vi "Wait for Acquisition Complete.vi"(8 "error in (no error)":errorcluster, 10 "Maximum Time (10000 ms)":i32=10000, 11 "VISA resource name":refnum<visa-resource-name>) -> (0 "error out":errorcluster, 3 "VISA resource name out":refnum<visa-resource-name>)   [LabVIEW 2018, in "Agilent U2000 Series.lvlib"]
doc: "Waits for the current acquisition to finish. This VI should be called after Initiate VI and before Fetch VI.\n\nNote:\nUse this VI only with other low-level VIs. The high-level VIs automatically incorporate this functionality. This VI does not check the instrument status."
uses:
  Agilent U2000 Series.lvlib
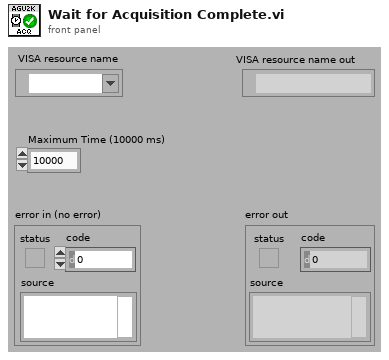
[diagram p1: front panel]
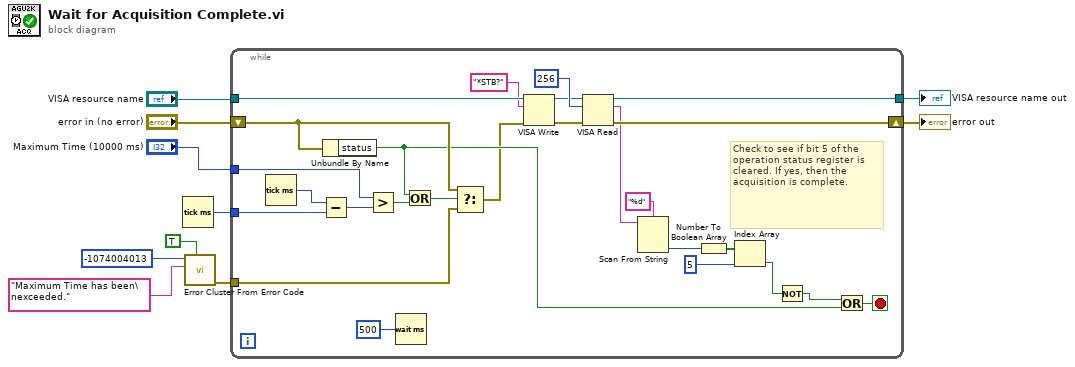
[diagram p0: block diagram]
diagram:
  n1 = Tick Count (ms)() -> (millisecond timer value=w4:u32)
  n2 = call <vilib>:"Error Cluster From Error Code.vi"("show call chain? (False)"=TRUE, "error message (\"\")"="Maximum Time has been\nexceeded." ("error message (\"\")"), "error code (0)"=-1074004013) -> ("error out"=w3:errorcluster)  [unwired: 1 in, 5 out]
  n3 = while {
    tunnel: [w35] -> w1
    tunnel: "VISA resource name" -> [w19]
    tunnel: "Maximum Time (10000 ms)" -> [w31]
    tunnel: w4 -> [w32]
    tunnel: w3 -> [w27]
    shift-right: [w36] -> w2
    shift-left: "error in (no error)" -> [w28]
    stop <- w26 stop-if-true
    # "Check to see if bit 5 of the operation status register is cleared. If yes, then the acquisition is complete."
    n4 = Tick Count (ms)() -> (millisecond timer value=w34:u32)
    n5 = Subtract(x=w34, y=w32) -> (x-y=w33:u32)
    n6 = Unbundle By Name(w28) -> ("status"=w25:bool)
    n7 = Greater?(x=w31, y=w33) -> (0:w30:bool)
    n8 = Wait (ms)(milliseconds to wait=u32 500) -> ()  [unwired: 1 out]
    n9 = Or(x=w25, y=w30) -> (x .or. y?=w29:bool)
    n10 = Select(t=w28, s=w29, f=w27) -> (s? t:f=w20:errorcluster)
    n11 = VISA Write(VISA resource name=w19, write buffer="*STB?", error in (no error)=w20) -> (VISA resource name out=w11:refnum<visa-resource-name>, error out=w12:errorcluster)  [unwired: 1 out]
    n12 = VISA Read(VISA resource name=w11, byte count=u32 256, error in (no error)=w12) -> (VISA resource name out=w35:refnum<visa-resource-name>, read buffer=w15:string, error out=w36:errorcluster)  [unwired: 1 out]
    n13 = Scan From String(format string="%d", input string=w15) -> (output 1=w21:i32)  [unwired: 3 in, 3 out]
    n14 = Number To Boolean Array(number=w21) -> (Boolean array=w24:bool[])
    n15 = Index Array(array=w24, index=5) -> (element=w18:bool)
    n16 = Not(x=w18) -> (.not. x?=w17:bool)
    n17 = Or(x=w17, y=w25) -> (x .or. y?=w26:bool)
  }
  "error out" <- w2
  "VISA resource name out" <- w1
